vi "Event Initialize.vi"(10 "Interactive Action":T1) -> (2 "User Event":refnum<user-event>, 3 "Event Reg Ref":refnum<event-registration>)   [LabVIEW 2018]
doc: "本VI是为《我和LabVIEW》一书编写的示例。\n关于本书的介绍请参考网页：\nhttp://ruanqizhen.spaces.live.com/blog/cns!5852D4F797C53FB6!4310.entry"
uses:
  Control/Interactive Action.ctl
  Othello.xctl
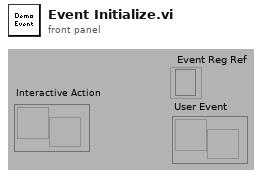
[diagram p1: front panel]
types:
  T1 = typedef "Othello.xctl/Interactive Action.ctl" = refnum<user-event>
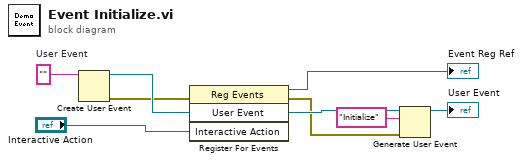
[diagram p0: block diagram]
diagram:
  w8 = ""  # User Event
  n1 = Create User Event(user event datatype=w8) -> (user event=w6:refnum<user-event>, error out=w1:errorcluster)  [unwired: 1 in]
  n2 = register-events(error in=w1, w6, "Interactive Action") -> (reference out=→"Event Reg Ref":refnum<event-registration>, error out=w4:errorcluster)  [unwired: 1 in]
  n3 = Generate User Event(user event=w6, event data cluster="Initialize" ("Event Name"), error in=w4) -> (user event out=→"User Event":refnum<user-event>)  [unwired: 1 in, 1 out]
